vi "RM.BuildRIODeviceTree.vi"(11 "deviceInfo array":T1[](array[typedef]) {"cd node ref" format="%.0x"}) -> (3 "RIO Device Tree Entries":T3(array[cluster]))   [LabVIEW 2016, in "FPGA Resource Manager.lvlib"]
uses:
  FPGA Resource Manager.lvlib
  RM.serverInfo.ctl
  <vilib>/NI Veristand/Custom Device API/Custom Device Item Ref.ctl
  <vilib>/NI Veristand/Custom Device API/Custom Device API.lvlib
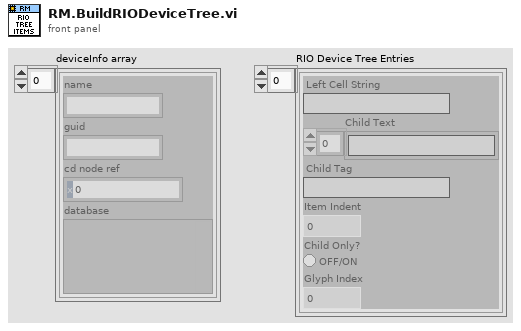
[diagram p1: front panel]
types:
  T1 = typedef "FPGA Resource Manager.lvlib/RM.serverInfo.ctl" = cluster{"name":string, "guid":string, "cd node ref":T2, "database":variant}
  T2 = typedef "Custom Device API.lvlib/Custom Device Item Ref.ctl" = u64
  T3 = cluster{"Left Cell String":string, "Child Text":string[], "Child Tag":string, "Item Indent":i32, "Child Only?":bool, "Glyph Index":i32}[]
  T4 = cluster{"Left Cell String":string, "Child Text":string[], "Child Tag":string, "Item Indent":i32, "Child Only?":bool, "Glyph Index":i32}
  T5 = typedef "FPGA Resource Manager.lvlib/RM.resourceType.ctl" = enum16{"Scalar Input", "Scalar Output", "Waveform Input", "Waveform Output"}
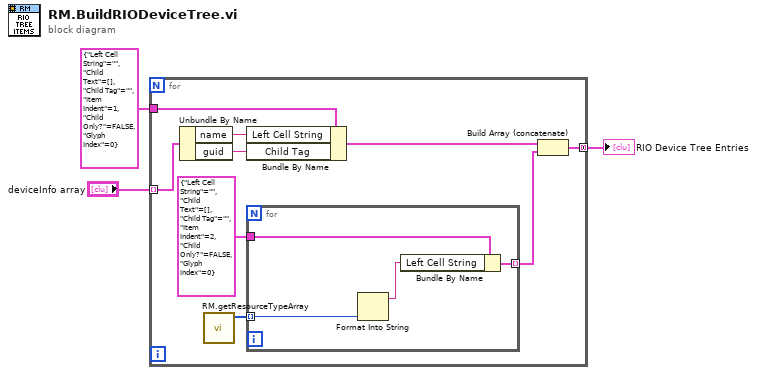
[diagram p0: block diagram]
diagram:
  n1 = for {
    tunnel: T4 {"Left Cell String"="", "Child Text"=[], "Child Tag"="", "Item Indent"=1, "Child Only?"=FALSE, "Glyph Index"=0} ("Item") -> [w12]
    tunnel: [w7] -> w3 mode=concatenating
    tunnel: "deviceInfo array" -> [w6] mode=indexing
    n2 = Unbundle By Name(w6) -> ("name"=w5:string, "guid"=w4:string)
    n3 = call "RM.getResourceTypeArray.vi"() -> ("Array"=w10:T5[])  [unwired: 11 in]
    n4 = Bundle By Name(cluster=w12, "Left Cell String"=w5, "Child Tag"=w4) -> (w11:T4)
    n5 = for {
      tunnel: w10 -> [w16] mode=indexing
      tunnel: T4 {"Left Cell String"="", "Child Text"=[], "Child Tag"="", "Item Indent"=2, "Child Only?"=FALSE, "Glyph Index"=0} ("Item") -> [w15]
      tunnel: [w14] -> w8 mode=indexing
      n6 = Format Into String(w16) -> (resulting string=w13:string)  [unwired: 3 in, 1 out]
      n7 = Bundle By Name(cluster=w15, "Left Cell String"=w13) -> (w14:T4)
    }
    n8 = Build Array (concatenate)(w11, w8) -> (w7:T3)
  }
  "RIO Device Tree Entries" <- w3
